vi "Read Configuration Class Name.vi"(8 "error in":errorcluster, 11 "TDMS datalogger editor node in":refnum<class "TDMS datalogger editor node.lvclass">) -> (0 "error out":errorcluster, 2 "Class Name":string, 3 "TDMS datalogger editor node out":refnum<class "TDMS datalogger editor node.lvclass">)   [LabVIEW 2013, in "TDMS datalogger editor node.lvclass"]
uses:
  TDMS datalogger editor node.lvclass
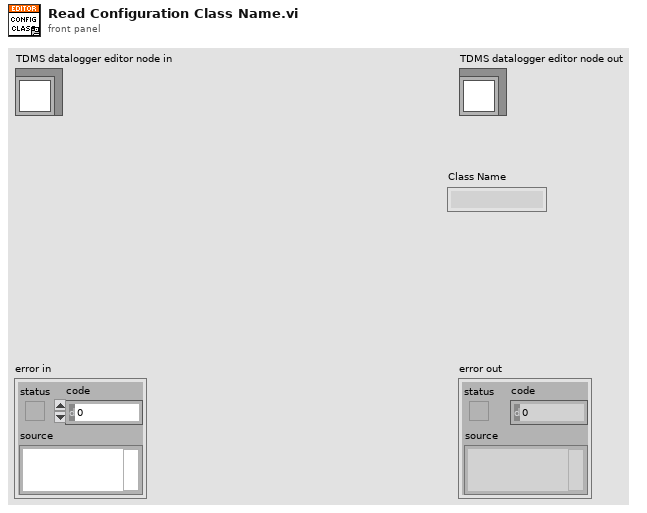
[diagram p1: front panel]
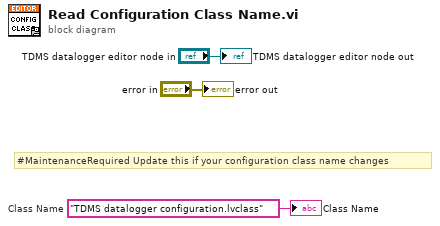
[diagram p0: block diagram]
diagram:
  w1 = "TDMS datalogger configuration.lvclass"  # Class Name
  # "#MaintenanceRequired Update this if your configuration class name changes"
  "error out" <- "error in"
  "TDMS datalogger editor node out" <- "TDMS datalogger editor node in"
  "Class Name" <- w1
